vi "Recloser_all.vi"() -> ()   [LabVIEW 2016]
uses:
  <vilib>/Utility/error.llb/DialogType.ctl
  <vilib>/FPGAPlugInAG/cRIO-9039 (Sync)/niLvFpga_Open_cRIO-9039 (Sync).vi
  <vilib>/rvi/interface/common/dynamic/niFpgaDynamicAddResources.vi
  <vilib>/Utility/error.llb/Error Cluster From Error Code.vi
  <vilib>/rvi/errors/niLvFpgaAdjustHostInterfaceError.vi
  <vilib>/FPGAPlugInAG/Dynamic/niLvFpga_Abort_Dynamic.vi
  <vilib>/FPGAPlugInAG/Dynamic/niLvFpga_Close_Dynamic.vi
  <vilib>/rvi/interface/nirviOpenFPGA/nirviOpenFPGA.xnode
  FPGA Bitfiles/IntelliRupter_calibrated.lvbitx
  <vilib>/rvi/interface/nirviReadWriteControl/nirviReadWriteControl.xnode
  <vilib>/rvi/interface/nirviMethod/nirviMethod.xnode
  <vilib>/rvi/interface/nirviCloseFPGA/nirviCloseFPGA.xnode
  <vilib>/rvi/interface/Simulation/niFpgaSimulationCallBeginRW.vi
  NiFpgaLv.dll
panel:
  out "error out":errorcluster
  out "Relay_toMGCC":bool[](array[boolean])
  out "Waveform Chart 3":dbl(graph)
  out "Counter Out":dbl
  out "Waveform Chart 2":dbl(graph)
  out "Waveform Chart":dbl(graph)
  out "magnitude difference 2":dbl
  out "frequency difference 2":dbl
  out "Phase difference 2":dbl
  out "Phase difference":dbl
  out "frequency difference":dbl
  out "magnitude difference":dbl
  in  "Relay8":bool
  in  "Relay7":bool
  in  "Relay6":bool
  in  "Relay5":bool
  in  "Relay4":bool
  in  "Relay3":bool
  in  "Relay2":bool
  in  "Relay1":bool
  in  "Recloser Settings":T1
  in  "samples per cycle":u16=192
  in  "Count(ticks)":u32=200
  in  "nominal frequency":u16=60
  out "basic calc interval":u16=38
  out "half cycle (samples)":i32=96
  in  "stop":bool
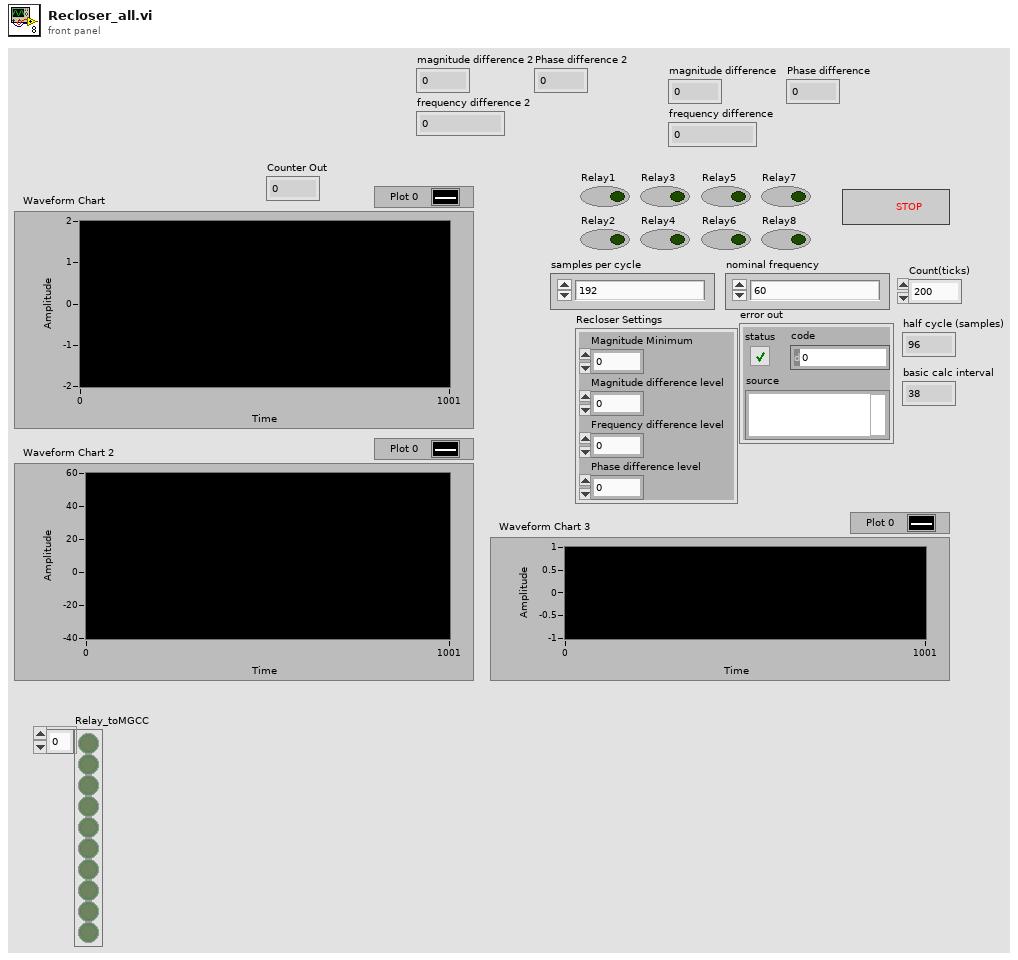
[diagram p1: front panel]
types:
  T1 = cluster{"Magnitude Minimum":dbl, "Magnitude difference level":dbl, "Frequency difference level":dbl, "Phase difference level":dbl}
  T2 = enum16{"Va L", "Vb L", "Vc L", "Ia", "Ib", "Ic", "Va R", "Vb R", "Vc R"}[]
  T3 = typedef "DialogType.ctl" = u16
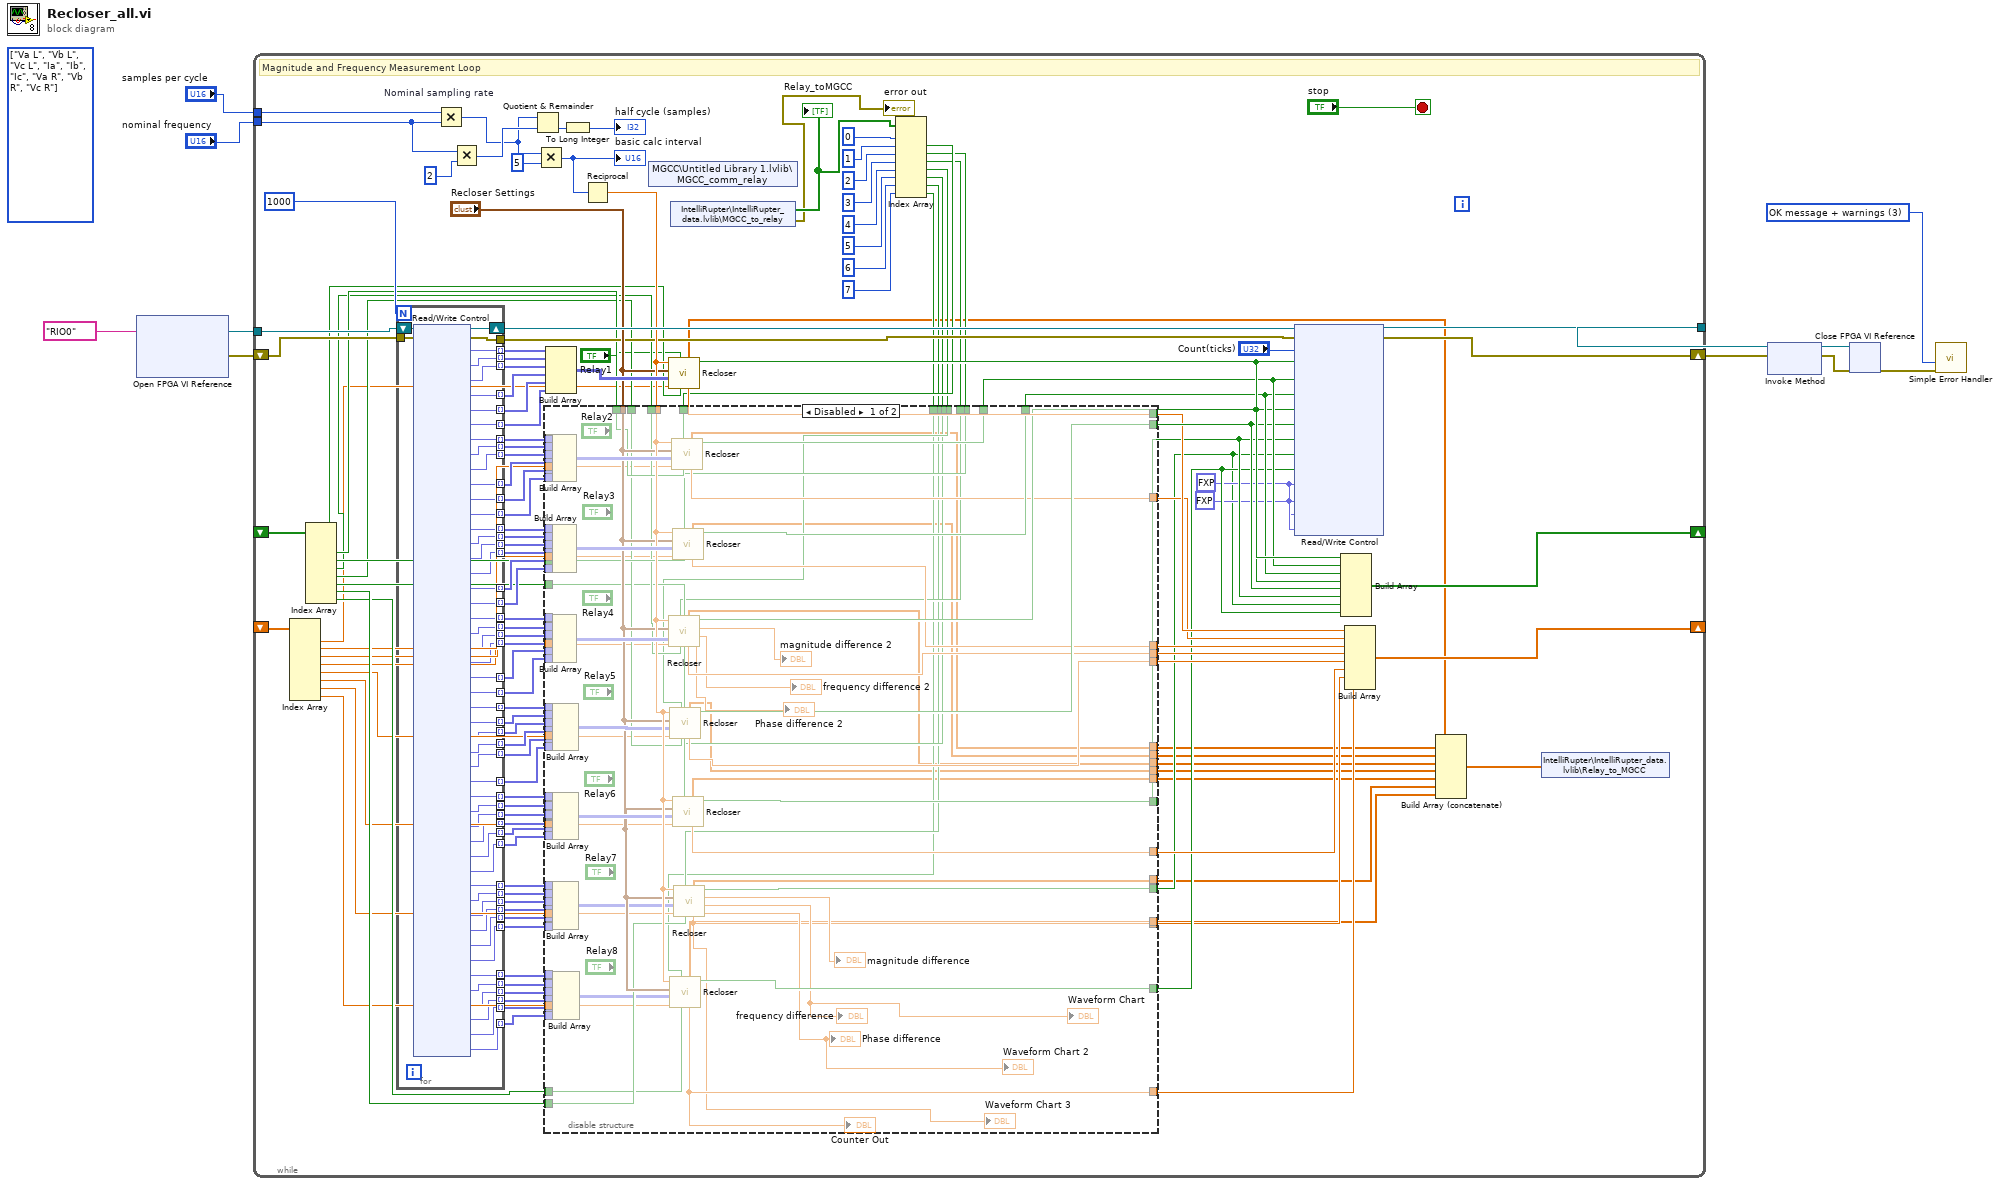
[diagram p0: block diagram]
diagram:
  (unwired) T2 [enum."Va L", enum."Vb L", enum."Vc L", enum."Ia", enum."Ib", enum."Ic", enum."Va R", enum."Vb R", enum."Vc R"] items=["Va L", "Vb L", "Vc L", "Ia", "Ib", "Ic", "Va R", "Vb R", "Vc R"] ("Enum")
  w10 = T3 3 items=["no dialog", "OK message", "continue or stop message", "OK message + warnings", "continue/stop + warnings"] ("type of dialog (OK msg:1)")
  n1 = xnode "Open FPGA VI Reference"("resource name"=tag "RIO0") -> ("FPGA VI Reference Out"=w3:refnum<k20>, "error out"=w4:errorcluster)  [unwired: 1 in]
  n2 = while {
    shift-right: [w77] -> w9
    shift-left: w4 -> [w79]
    tunnel: w3 -> [w136]
    tunnel: [w134] -> w8
    tunnel: "samples per cycle" -> [w145]
    tunnel: "nominal frequency" -> [w144]
    shift-right: [w71] -> _
    shift-left: _ -> [w70]
    shift-right: [w53] -> _
    shift-left: _ -> [w52]
    stop <- "stop" stop-if-true
    w42 = fxp<+/-,52,10> 0.0 ("I offset")
    w41 = fxp<+/-,26,5> 1.0 ("I scale factor")
    # "Magnitude and Frequency Measurement Loop"
    n3 = Index Array(array=w52) -> (element #1=w51:dbl, element #2=w50:dbl, element #3=w49:dbl, element #4=w48:dbl, element #5=w47:dbl, element #6=w46:dbl, element #7=w45:dbl, element #8=w44:dbl)  [unwired: 8 in]
    n4 = Index Array(array=w70) -> (element #1=w69:bool, element #2=w68:bool, element #3=w67:bool, element #4=w66:bool, element #5=w65:bool, element #6=w64:bool, element #7=w63:bool, element #8=w62:bool)  [unwired: 8 in]
    n5 = for {
      N: 1000 -> [_]
      tunnel: [w294] -> w133 mode=indexing
      tunnel: [w293] -> w132 mode=indexing
      tunnel: [w292] -> w131 mode=indexing
      tunnel: [w291] -> w130 mode=indexing
      tunnel: [w290] -> w129 mode=indexing
      tunnel: [w289] -> w128 mode=indexing
      tunnel: [w288] -> w127 mode=indexing
      tunnel: [w287] -> w126 mode=indexing
      tunnel: [w286] -> w125 mode=indexing
      tunnel: [w285] -> w124 mode=indexing
      tunnel: [w284] -> w123 mode=indexing
      tunnel: [w283] -> w122 mode=indexing
      tunnel: [w282] -> w121 mode=indexing
      tunnel: [w281] -> w120 mode=indexing
      tunnel: [w280] -> w119 mode=indexing
      tunnel: [w279] -> w118 mode=indexing
      tunnel: [w278] -> w117 mode=indexing
      tunnel: [w277] -> w116 mode=indexing
      tunnel: [w276] -> w115 mode=indexing
      tunnel: [w275] -> w114 mode=indexing
      tunnel: [w274] -> w113 mode=indexing
      tunnel: [w273] -> w112 mode=indexing
      tunnel: [w272] -> w111 mode=indexing
      tunnel: [w271] -> w110 mode=indexing
      shift-right: [w295] -> w135
      shift-left: w136 -> [w296]
      tunnel: [w270] -> w108 mode=indexing
      tunnel: [w269] -> w107 mode=indexing
      tunnel: [w268] -> w106 mode=indexing
      tunnel: [w267] -> w105 mode=indexing
      tunnel: [w266] -> w104 mode=indexing
      tunnel: [w265] -> w103 mode=indexing
      tunnel: [w264] -> w102 mode=indexing
      tunnel: [w263] -> w101 mode=indexing
      tunnel: [w262] -> w100 mode=indexing
      tunnel: [w261] -> w99 mode=indexing
      tunnel: [w260] -> w98 mode=indexing
      tunnel: [w259] -> w97 mode=indexing
      tunnel: [w258] -> w96 mode=indexing
      tunnel: [w257] -> w95 mode=indexing
      tunnel: [w256] -> w94 mode=indexing
      tunnel: [w255] -> w93 mode=indexing
      tunnel: [w254] -> w92 mode=indexing
      tunnel: [w253] -> w91 mode=indexing
      tunnel: [w252] -> w90 mode=indexing
      tunnel: [w251] -> w89 mode=indexing
      tunnel: [w250] -> w88 mode=indexing
      tunnel: [w249] -> w87 mode=indexing
      tunnel: [w248] -> w86 mode=indexing
      tunnel: [w247] -> w85 mode=indexing
      tunnel: w79 -> [w246]
      tunnel: [w245] -> w78
      n6 = xnode "Read/Write Control"("FPGA VI Reference In"=w296, "error in"=w246) -> ("FPGA VI Reference Out"=w295:refnum<k20>, "error out"=w245:errorcluster, "V1L AB"=w288:fxp<+/-,53,11>, "V1L BC"=w287:fxp<+/-,53,11>, "V1L CA"=w286:fxp<+/-,53,11>, "V1R AB"=w285:fxp<+/-,53,11>, "V1R BC"=w284:fxp<+/-,53,11>, "V1R CA"=w283:fxp<+/-,53,11>, "V2L AB"=w294:fxp<+/-,53,11>, "V2L BC"=w293:fxp<+/-,53,11>, "V2L CA"=w292:fxp<+/-,53,11>, "V2R AB"=w291:fxp<+/-,53,11>, "V2R BC"=w290:fxp<+/-,53,11>, "V2R CA"=w289:fxp<+/-,53,11>, "V3L AB"=w282:fxp<+/-,53,11>, "V3L BC"=w281:fxp<+/-,53,11>, "V3L CA"=w280:fxp<+/-,53,11>, "V3R AB"=w279:fxp<+/-,53,11>, "V3R BC"=w278:fxp<+/-,53,11>, "V3R CA"=w277:fxp<+/-,53,11>, "V4L AB"=w276:fxp<+/-,53,11>, "V4L BC"=w275:fxp<+/-,53,11>, "V4L CA"=w274:fxp<+/-,53,11>, "V4R AB"=w273:fxp<+/-,53,11>, "V4R BC"=w272:fxp<+/-,53,11>, "V4R CA"=w271:fxp<+/-,53,11>, "V5L AB"=w270:fxp<+/-,53,11>, "V5L BC"=w269:fxp<+/-,53,11>, "V5L CA"=w268:fxp<+/-,53,11>, "V5R AB"=w267:fxp<+/-,53,11>, "V5R BC"=w266:fxp<+/-,53,11>, "V5R CA"=w265:fxp<+/-,53,11>, "V6L AB"=w264:fxp<+/-,53,11>, "V6L BC"=w263:fxp<+/-,53,11>, "V6L CA"=w262:fxp<+/-,53,11>, "V6R AB"=w261:fxp<+/-,53,11>, "V6R BC"=w260:fxp<+/-,53,11>, "V6R CA"=w259:fxp<+/-,53,11>, "V7L AB"=w258:fxp<+/-,53,11>, "V7L BC"=w257:fxp<+/-,53,11>, "V7L CA"=w256:fxp<+/-,53,11>, "V7R AB"=w255:fxp<+/-,53,11>, "V7R BC"=w254:fxp<+/-,53,11>, "V7R CA"=w253:fxp<+/-,53,11>, "V8L AB"=w252:fxp<+/-,53,11>, "V8L BC"=w251:fxp<+/-,53,11>, "V8L CA"=w250:fxp<+/-,53,11>, "V8R AB"=w249:fxp<+/-,53,11>, "V8R BC"=w248:fxp<+/-,53,11>, "V8R CA"=w247:fxp<+/-,53,11>)
    }
    n7 = Multiply "Nominal sampling rate"(x=w145, y=w144) -> (x*y=w137:u16)
    n8 = Multiply(x=w144, y=2) -> (x*y=w142:i32)
    n9 = Quotient & Remainder(x=w137, y=w142) -> (floor(x/y)=w140:i32)  [unwired: 1 out]
    n10 = Multiply(x=w137, y=u16 5) -> (x*y=w84:u16)
    "basic calc interval" <- w84
    n11 = Build Array(w127, w126, w125, w124, w123, w122) -> (w82:fxp<+/-,53,11>[][])
    n12 = To Long Integer(number=w140) -> (32bit integer=→"half cycle (samples)":i32)
    n13 = Reciprocal(x=w84) -> (1/x=w81:dbl)
    n14 = shared-variable "MGCC\\Untitled Library 1.lvlib\\MGCC_comm_relay"() -> ()  [unwired: 1 in, 2 out]
    n15 = call "Recloser.vi"("Current state"=w69, "Relay"="Relay1", "Counter In"=w51, "Input array"=w82, "Recloser Settings"="Recloser Settings", "dt"=w81) -> ("Recloser action"=w76:bool, "Counter Out"=w61:dbl, "Combined data for communication"=w21:dbl[])  [unwired: 3 out]
    n16 = shared-variable "IntelliRupter\\IntelliRupter_data.lvlib\\MGCC_to_relay"() -> (w23:bool[], error out=→"error out":errorcluster)  [unwired: 1 in]
    "Relay_toMGCC" <- w23
    n17 = Index Array(array=w23, index #1=0 ("index"), index #2=1 ("index"), index #3=2 ("index"), index #4=3 ("index"), index #5=4 ("index"), index #6=5 ("index"), index #7=6 ("index"), index #8=7 ("index")) -> (element #2=w30:bool, element #3=w29:bool, element #4=w28:bool, element #5=w27:bool, element #6=w26:bool, element #7=w25:bool, element #8=w24:bool)  [unwired: 1 out]
    n18 = disable-structure shown="Disabled" {
      disable-tunnel: w133 -> [w244 _]
      disable-tunnel: w132 -> [w243 _]
      disable-tunnel: w131 -> [w242 _]
      disable-tunnel: w130 -> [w241 _]
      disable-tunnel: w129 -> [w240 _]
      disable-tunnel: w128 -> [w239 _]
      disable-tunnel: w121 -> [w238 _]
      disable-tunnel: w120 -> [w237 _]
      disable-tunnel: w119 -> [w236 _]
      disable-tunnel: w118 -> [w235 _]
      disable-tunnel: w117 -> [w234 _]
      disable-tunnel: w116 -> [w233 _]
      disable-tunnel: w115 -> [w232 _]
      disable-tunnel: w114 -> [w231 _]
      disable-tunnel: w113 -> [w230 _]
      disable-tunnel: w112 -> [w229 _]
      disable-tunnel: w111 -> [w228 _]
      disable-tunnel: w110 -> [w227 _]
      disable-tunnel: w108 -> [w226 _]
      disable-tunnel: w107 -> [w225 _]
      disable-tunnel: w106 -> [w224 _]
      disable-tunnel: w105 -> [w223 _]
      disable-tunnel: w104 -> [w222 _]
      disable-tunnel: w103 -> [w221 _]
      disable-tunnel: w102 -> [w220 _]
      disable-tunnel: w101 -> [w219 _]
      disable-tunnel: w100 -> [w218 _]
      disable-tunnel: w99 -> [w217 _]
      disable-tunnel: w98 -> [w216 _]
      disable-tunnel: w97 -> [w215 _]
      disable-tunnel: w96 -> [w214 _]
      disable-tunnel: w95 -> [w213 _]
      disable-tunnel: w94 -> [w212 _]
      disable-tunnel: w93 -> [w211 _]
      disable-tunnel: w92 -> [w210 _]
      disable-tunnel: w91 -> [w209 _]
      disable-tunnel: w90 -> [w208 _]
      disable-tunnel: w89 -> [w207 _]
      disable-tunnel: w88 -> [w206 _]
      disable-tunnel: w87 -> [w205 _]
      disable-tunnel: w86 -> [w204 _]
      disable-tunnel: w85 -> [w203 _]
      disable-tunnel: w81 -> [w199 _]
      disable-tunnel: "Recloser Settings" -> [w196 _]
      disable-tunnel: [w195 _] -> w75
      disable-tunnel: [w194 _] -> w74
      disable-tunnel: [w193 _] -> w73
      disable-tunnel: [w192 _] -> w72
      disable-tunnel: w68 -> [w191 _]
      disable-tunnel: w67 -> [w190 _]
      disable-tunnel: w66 -> [w189 _]
      disable-tunnel: w65 -> [w188 _]
      disable-tunnel: w64 -> [w187 _]
      disable-tunnel: w63 -> [w186 _]
      disable-tunnel: w62 -> [w185 _]
      disable-tunnel: [w184 _] -> w60
      disable-tunnel: [w183 _] -> w59
      disable-tunnel: [w182 _] -> w58
      disable-tunnel: [w181 _] -> w57
      disable-tunnel: [w180 _] -> w56
      disable-tunnel: [w179 _] -> w55
      disable-tunnel: [w178 _] -> w54
      disable-tunnel: w50 -> [w177 _]
      disable-tunnel: w49 -> [w176 _]
      disable-tunnel: w48 -> [w175 _]
      disable-tunnel: w47 -> [w174 _]
      disable-tunnel: w46 -> [w173 _]
      disable-tunnel: w45 -> [w172 _]
      disable-tunnel: w44 -> [w171 _]
      disable-tunnel: [w167 _] -> w43
      disable-tunnel: [w161 _] -> w40
      disable-tunnel: [w160 _] -> w39
      disable-tunnel: w30 -> [w159 _]
      disable-tunnel: w29 -> [w158 _]
      disable-tunnel: w28 -> [w157 _]
      disable-tunnel: w27 -> [w156 _]
      disable-tunnel: w26 -> [w155 _]
      disable-tunnel: w25 -> [w154 _]
      disable-tunnel: w24 -> [w153 _]
      disable-tunnel: [w152 _] -> w20
      disable-tunnel: [w151 _] -> w18
      disable-tunnel: [w150 _] -> w17
      disable-tunnel: [w149 _] -> w16
      disable-tunnel: [w148 _] -> w15
      disable-tunnel: [w147 _] -> w14
      disable-tunnel: [w146 _] -> w13
      frame Disabled {
        n19 = Build Array(w244, w243, w242, w241, w240, w239) -> (w202:fxp<+/-,53,11>[][])
        n20 = Build Array(w238, w237, w236, w235, w234, w233) -> (w201:fxp<+/-,53,11>[][])
        n21 = Build Array(w232, w231, w230, w229, w228, w227) -> (w200:fxp<+/-,53,11>[][])
        n22 = Build Array(w226, w225, w224, w223, w222, w221) -> (w198:fxp<+/-,53,11>[][])
        n23 = Build Array(w220, w219, w218, w217, w216, w215) -> (w197:fxp<+/-,53,11>[][])
        n24 = Build Array(w214, w213, w212, w211, w210, w209) -> (w166:fxp<+/-,53,11>[][])
        n25 = Build Array(w208, w207, w206, w205, w204, w203) -> (w165:fxp<+/-,53,11>[][])
        n26 = call "Recloser.vi"("Current state"=w189, "Relay"=w157, "Counter In"=w175, "Input array"=w200, "Recloser Settings"=w196, "dt"=w199) -> ("Phase difference"=→"Phase difference 2":dbl, "frequency difference"=→"frequency difference 2":dbl, "magnitude difference"=→"magnitude difference 2":dbl, "Recloser action"=w193:bool, "Counter Out"=w182:dbl, "Combined data for communication"=w150:dbl[])
        n27 = call "Recloser.vi"("Current state"=w188, "Relay"=w156, "Counter In"=w174, "Input array"=w198, "Recloser Settings"=w196, "dt"=w199) -> ("Recloser action"=w192:bool, "Counter Out"=w181:dbl, "Combined data for communication"=w149:dbl[])  [unwired: 3 out]
        n28 = call "Recloser.vi"("Current state"=w185, "Relay"=w153, "Counter In"=w171, "Input array"=w165, "Recloser Settings"=w196, "dt"=w199) -> ("Recloser action"=w178:bool, "Counter Out"=w167:dbl, "Combined data for communication"=w146:dbl[])  [unwired: 3 out]
        "Counter Out" <- w167
        n29 = call "Recloser.vi"("Current state"=w191, "Relay"=w159, "Counter In"=w177, "Input array"=w202, "Recloser Settings"=w196, "dt"=w199) -> ("Recloser action"=w195:bool, "Counter Out"=w184:dbl, "Combined data for communication"=w152:dbl[])  [unwired: 3 out]
        n30 = call "Recloser.vi"("Current state"=w190, "Relay"=w158, "Counter In"=w176, "Input array"=w201, "Recloser Settings"=w196, "dt"=w199) -> ("Recloser action"=w194:bool, "Counter Out"=w183:dbl, "Combined data for communication"=w151:dbl[])  [unwired: 3 out]
        n31 = call "Recloser.vi"("Current state"=w187, "Relay"=w155, "Counter In"=w173, "Input array"=w197, "Recloser Settings"=w196, "dt"=w199) -> ("Recloser action"=w179:bool, "Counter Out"=w180:dbl, "Combined data for communication"=w148:dbl[])  [unwired: 3 out]
        n32 = call "Recloser.vi"("Current state"=w186, "Relay"=w154, "Counter In"=w172, "Input array"=w166, "Recloser Settings"=w196, "dt"=w199) -> ("Phase difference"=→"Phase difference" →"Waveform Chart 2":dbl, "frequency difference"=→"frequency difference" →"Waveform Chart":dbl, "magnitude difference"=→"magnitude difference":dbl, "Recloser action"=w161:bool, "Counter Out"=w160:dbl, "Combined data for communication"=w147:dbl[])
        "Waveform Chart 3" <- w160
      }
      frame Enabled {
      }
    }
    n33 = xnode "Read/Write Control"("FPGA VI Reference In"=w135, "error in"=w78, "Count(ticks)"="Count(ticks)", "Relay1"=w76, "Relay2"=w75, "Relay3"=w74, "Relay4"=w73, "Relay5"=w72, "Relay6"=w55, "Relay7"=w40, "Relay8"=w54, "I scale factor"=w41, "I offset"=w42, "V scale factor"=w41, "V offset"=w42) -> ("FPGA VI Reference Out"=w134:refnum<k20>, "error out"=w77:errorcluster)
    n34 = Build Array(w76, w75, w74, w73, w72, w55, w40, w54) -> (w71:bool[])
    n35 = Build Array(w61, w60, w59, w58, w57, w56, w39, w43) -> (w53:dbl[])
    n36 = Build Array (concatenate)(w21, w20, w18, w17, w16, w15, w14, w13) -> (w19:dbl[])
    n37 = shared-variable "IntelliRupter\\IntelliRupter_data.lvlib\\Relay_to_MGCC"(w19) -> ()  [unwired: 1 in, 1 out]
  }
  n38 = xnode "Invoke Method"("FPGA VI Reference In"=w8, "error in"=w9) -> ("FPGA VI Reference Out"=w7:refnum<k20>, "error out"=w6:errorcluster)
  n39 = xnode "Close FPGA VI Reference"("FPGA VI Reference In"=w7, "error in"=w6) -> ("error out"=w11:errorcluster)
  n40 = call <vilib>:"Simple Error Handler.vi"("type of dialog (OK msg:1)"=w10, "error in (no error)"=w11) -> ()  [unwired: 3 in, 5 out]
